vi "Destroy Stream Events.vi"(8 "error in (no error)":errorcluster, 11 "Stream User Events":T1) -> (0 "error out":errorcluster)   [LabVIEW 2020, in "Camera.lvclass"]
uses:
  Camera.lvclass
  Stream User Events.ctl
  Camera.lvclass/Camera.ctl
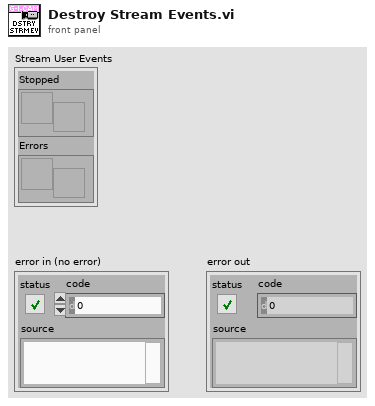
[diagram p1: front panel]
types:
  T1 = typedef "Camera.lvclass/Stream User Events.ctl" = cluster{"Stopped":refnum<user-event>, "Errors":refnum<user-event>}
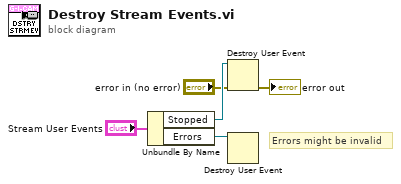
[diagram p0: block diagram]
diagram:
  # "Errors might be invalid"
  n1 = Unbundle By Name("Stream User Events") -> ("Stopped"=w4:refnum<user-event>, "Errors"=w5:refnum<user-event>)
  n2 = Destroy User Event(user event=w4, error in="error in (no error)") -> (error out=→"error out":errorcluster)
  n3 = Destroy User Event(user event=w5) -> ()  [unwired: 1 in, 1 out]
